vi "ConfiguracaoPortaDAQ.vi"(8 "error in":errorcluster, 11 "AnalogTasksConfiguration":string[][](array[string])) -> (0 "error out":errorcluster, 2 "Info":string[](array[string]), 3 "AnalogTasks":cluster{"Function":i32, "Task":refnum<k21>}[](array[cluster]))   [LabVIEW 2019]
uses:
  <vilib>/DAQmx/create/channels.llb/DAQmx Create Channel (AI-Voltage-Basic).vi
  <vilib>/DAQmx/configure/timing.llb/DAQmx Timing (Sample Clock).vi
  <resource>/objmgr/daqmx.rc
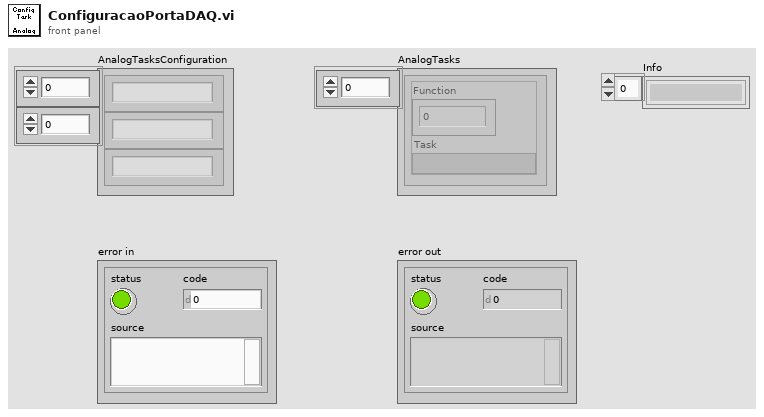
[diagram p1: front panel]
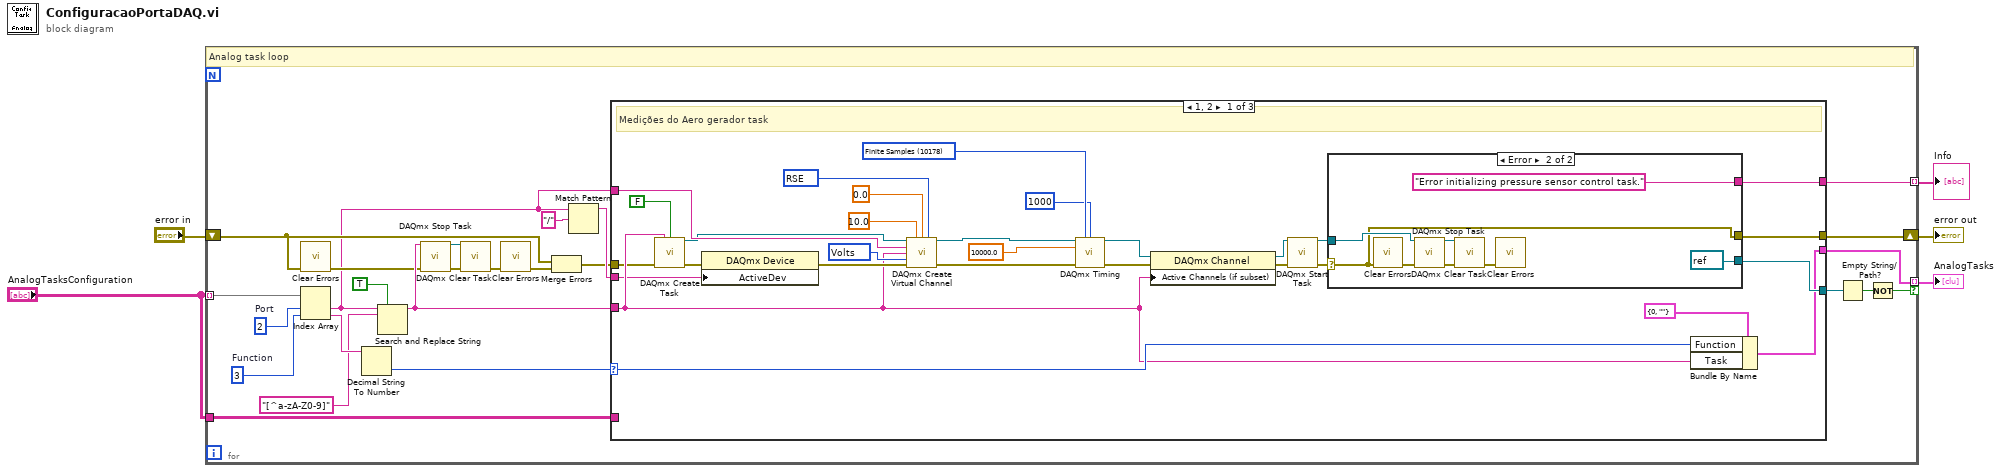
[diagram p0: block diagram]
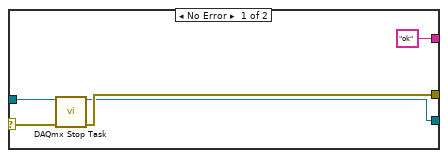
[diagram p2: hidden frame]
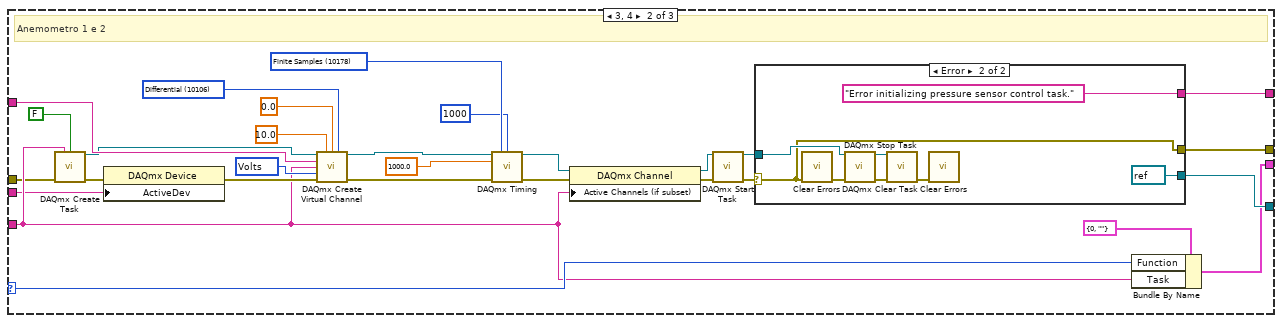
[diagram p3: hidden frame]
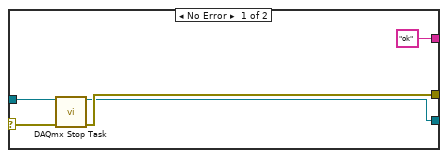
[diagram p4: hidden frame]
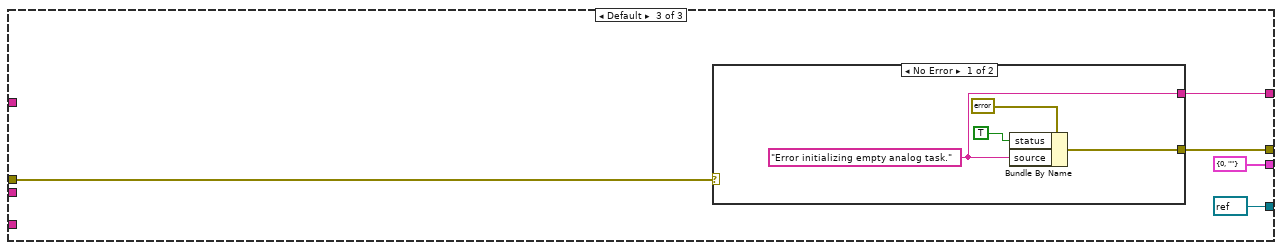
[diagram p5: hidden frame]
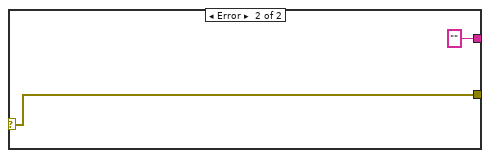
[diagram p6: hidden frame]
diagram:
  n1 = for {
    tunnel: "AnalogTasksConfiguration" -> [w29] mode=indexing
    shift-right: [w23] -> w5
    shift-left: "error in" -> [w19]
    tunnel: [w25] -> w4 mode=indexing if=w26
    tunnel: "AnalogTasksConfiguration" -> [w7]
    tunnel: [w6] -> w1 mode=indexing
    w28 = 3  # Function
    w30 = 2  # Port
    # "Analog task loop"
    n2 = call <vilib>:"Clear Errors.vi"("error in (no error)"=w19) -> ("error out"=w16:errorcluster)  [unwired: 5 in, 1 out]
    n3 = Index Array(array=w29, index #1=w30, index #2=w28) -> (element #1=w15:string, element #2=w18:string)
    n4 = Decimal String To Number(string=w18) -> (number=w17:i32)  [unwired: 2 in, 1 out]
    n5 = Search and Replace String(replace all?=TRUE ("replace all? (F)"), input string=w15, search string="[^a-zA-Z0-9]") -> (result string=w20:string)  [unwired: 5 in, 3 out]
    n6 = call <vilib>:"DAQmx Stop Task.vi"("task/channels in"=w20, "error in"=w16) -> ("task out"=w9:refnum<k21>, "error out"=w8:errorcluster)  [unwired: 12 in]
    n7 = call <vilib>:"DAQmx Clear Task.vi"("task in"=w9, "error in"=w8) -> ("error out"=w10:errorcluster)  [unwired: 13 in]
    n8 = call <vilib>:"Clear Errors.vi"("error in (no error)"=w10) -> ("error out"=w11:errorcluster)  [unwired: 5 in, 1 out]
    n9 = Merge Errors(w19, w11) -> (w21:errorcluster)
    n10 = Match Pattern(string=w15, regular expression="/") -> (before substring=w22:string)  [unwired: 1 in, 3 out]
    n11 = case shown="1, 2" w17 {
      selector: w17 -> [w51 w93 _]
      tunnel: [w54 w96 w116] -> w23
      tunnel: [w52 w94 refnum<k21> refnum ("task out")] -> w24
      tunnel: w21 -> [w47 w89 w117]
      tunnel: w15 -> [w57 w99 _]
      tunnel: w20 -> [w49 w91 _]
      tunnel: [w50 w92 cluster{"Function":i32, "Task":refnum<k21>} {"Function"=0, "Task"=""} ("TemporaryTask")] -> w25
      tunnel: w22 -> [w48 w90 _]
      tunnel: w7 -> [_ _ _]
      tunnel: [w33 w75 w115] -> w6
      frame 1, 2 {
        w38 = 10178 items=["Finite Samples"=10178, "Continuous Samples"=10123, "Hardware Timed Single Point"=12522] ("sample mode")
        w43 = 10083 items=["Default"=-1, "RSE"=10083, "NRSE"=10078, "Differential"=10106, "Pseudodifferential"=12529] ("input terminal configuration")
        w59 = 10348 items=["Volts"=10348, "From Custom Scale"=10065] ("units")
        # "Medições do Aero gerador task"
        n12 = call <vilib>:"DAQmx Create Task.vi"("new task name"=w49, "auto cleanup"=FALSE, "error in"=w47) -> ("task out"=w46:refnum<k21>, "error out"=w55:errorcluster)  [unwired: 11 in]
        n13 = property class="DAQmx Device"(error in=w55, "ActiveDev"=w48) -> (error out=w58:errorcluster)  [unwired: 1 in, 1 out]
        n14 = call-poly <vilib>:"DAQmx Create Virtual Channel.vi"("task in"=w46, "maximum value"=10.0, "minimum value"=0.0, "input terminal configuration"=w43, "physical channels"=w57, "name to assign"=w49, "units"=w59, "error in"=w58) -> ("task out"=w35:refnum<k21>, "error out"=w37:errorcluster)  [unwired: 6 in]
        n15 = call-poly <vilib>:"DAQmx Timing.vi"("task/channels in"=w35, "sample mode"=w38, "samples per channel"=1000, "rate"=10000.0, "error in"=w37) -> ("task out"=w34:refnum<k21>, "error out"=w36:errorcluster)  [unwired: 9 in]
        n16 = property class="DAQmx Channel"(reference=w34, error in=w36, "Active Channels (if subset)"=w49) -> (reference out=w42:refnum<k21>, error out=w40:errorcluster)
        n17 = call <vilib>:"DAQmx Start Task.vi"("task/channels in"=w42, "error in"=w40) -> ("task out"=w41:refnum<k21>, "error out"=w39:errorcluster)  [unwired: 12 in]
        n18 = case shown="Error" w39 {
          selector: w39 -> [w64 w65]
          tunnel: [w61 refnum<k21> refnum ("task in")] -> w52
          tunnel: w41 -> [w62 w72]
          tunnel: [w63 w65] -> w54
          tunnel: ["ok" ("Texto") "Error initializing pressure sensor control task." ("Texto")] -> w33
          frame No Error {
            n19 = call <vilib>:"DAQmx Stop Task.vi"("task/channels in"=w62, "error in"=w64) -> ("task out"=w61:refnum<k21>, "error out"=w63:errorcluster)  [unwired: 12 in]
          }
          frame Error {
            n20 = call <vilib>:"Clear Errors.vi"("error in (no error)"=w65) -> ("error out"=w68:errorcluster)  [unwired: 5 in, 1 out]
            n21 = call <vilib>:"DAQmx Stop Task.vi"("task/channels in"=w72, "error in"=w68) -> ("task out"=w70:refnum<k21>, "error out"=w71:errorcluster)  [unwired: 12 in]
            n22 = call <vilib>:"DAQmx Clear Task.vi"("task in"=w70, "error in"=w71) -> ("error out"=w67:errorcluster)  [unwired: 13 in]
            n23 = call <vilib>:"Clear Errors.vi"("error in (no error)"=w67) -> ()  [unwired: 5 in, 2 out]
          }
        }
        n24 = Bundle By Name(cluster=cluster{"Function":i32, "Task":refnum<k21>} {"Function"=0, "Task"=""} ("TemporaryTask"), "Function"=w51, "Task"=w49) -> (w50:cluster{"Function":i32, "Task":refnum<k21>})
      }
      frame 3, 4 {
        w80 = 10178 items=["Finite Samples"=10178, "Continuous Samples"=10123, "Hardware Timed Single Point"=12522] ("sample mode")
        w85 = 10106 items=["Default"=-1, "RSE"=10083, "NRSE"=10078, "Differential"=10106, "Pseudodifferential"=12529] ("input terminal configuration")
        w101 = 10348 items=["Volts"=10348, "From Custom Scale"=10065] ("units")
        # "Anemometro 1 e 2"
        n25 = call <vilib>:"DAQmx Create Task.vi"("new task name"=w91, "auto cleanup"=FALSE, "error in"=w89) -> ("task out"=w88:refnum<k21>, "error out"=w97:errorcluster)  [unwired: 11 in]
        n26 = property class="DAQmx Device"(error in=w97, "ActiveDev"=w90) -> (error out=w100:errorcluster)  [unwired: 1 in, 1 out]
        n27 = call-poly <vilib>:"DAQmx Create Virtual Channel.vi"("task in"=w88, "maximum value"=10.0, "minimum value"=0.0, "input terminal configuration"=w85, "physical channels"=w99, "name to assign"=w91, "units"=w101, "error in"=w100) -> ("task out"=w77:refnum<k21>, "error out"=w79:errorcluster)  [unwired: 6 in]
        n28 = call-poly <vilib>:"DAQmx Timing.vi"("task/channels in"=w77, "sample mode"=w80, "samples per channel"=1000, "rate"=1000.0, "error in"=w79) -> ("task out"=w76:refnum<k21>, "error out"=w78:errorcluster)  [unwired: 9 in]
        n29 = property class="DAQmx Channel"(reference=w76, error in=w78, "Active Channels (if subset)"=w91) -> (reference out=w84:refnum<k21>, error out=w82:errorcluster)
        n30 = call <vilib>:"DAQmx Start Task.vi"("task/channels in"=w84, "error in"=w82) -> ("task out"=w83:refnum<k21>, "error out"=w81:errorcluster)  [unwired: 12 in]
        n31 = case shown="Error" w81 {
          selector: w81 -> [w106 w107]
          tunnel: [w103 refnum<k21> refnum ("task in")] -> w94
          tunnel: w83 -> [w104 w114]
          tunnel: [w105 w107] -> w96
          tunnel: ["ok" ("Texto") "Error initializing pressure sensor control task." ("Texto")] -> w75
          frame No Error {
            n32 = call <vilib>:"DAQmx Stop Task.vi"("task/channels in"=w104, "error in"=w106) -> ("task out"=w103:refnum<k21>, "error out"=w105:errorcluster)  [unwired: 12 in]
          }
          frame Error {
            n33 = call <vilib>:"Clear Errors.vi"("error in (no error)"=w107) -> ("error out"=w110:errorcluster)  [unwired: 5 in, 1 out]
            n34 = call <vilib>:"DAQmx Stop Task.vi"("task/channels in"=w114, "error in"=w110) -> ("task out"=w112:refnum<k21>, "error out"=w113:errorcluster)  [unwired: 12 in]
            n35 = call <vilib>:"DAQmx Clear Task.vi"("task in"=w112, "error in"=w113) -> ("error out"=w109:errorcluster)  [unwired: 13 in]
            n36 = call <vilib>:"Clear Errors.vi"("error in (no error)"=w109) -> ()  [unwired: 5 in, 2 out]
          }
        }
        n37 = Bundle By Name(cluster=cluster{"Function":i32, "Task":refnum<k21>} {"Function"=0, "Task"=""} ("TemporaryTask"), "Function"=w93, "Task"=w91) -> (w92:cluster{"Function":i32, "Task":refnum<k21>})
      }
      frame Default {
        n38 = case shown="No Error" w117 {
          selector: w117 -> [_ w125]
          tunnel: [w122 w125] -> w116
          tunnel: [w120 "" ("Texto")] -> w115
          frame No Error {
            w120 = "Error initializing empty analog task." ("Texto")
            n39 = Bundle By Name(cluster=errorcluster {"status"=FALSE, "code"=0, "source"=""} ("error IO"), "status"=TRUE, "source"=w120) -> (w122:errorcluster)
          }
          frame Error {
          }
        }
      }
    }
    n40 = Empty String/Path?(string/path=w24) -> (empty?=w27:bool)
    n41 = Not(x=w27) -> (.not. x?=w26:bool)
  }
  "error out" <- w5
  "AnalogTasks" <- w4
  "Info" <- w1
